vi "createQueryInputStr.vi"(8 "error in (no error)":errorcluster, 9 "CoolerQuery":T1=enum."ReadControlSensor", 11 "CoolerSerialCommand in":refnum<class "CoolerSerialCommand.lvclass">) -> (0 "error out":errorcluster, 2 "cmdDataStr":string, 3 "CoolerSerialCommand out":refnum<class "CoolerSerialCommand.lvclass">)   [LabVIEW 2016, in "CoolerSerialCommand.lvclass"]
uses:
  CoolerSerialCommand.lvclass
  typedefs/CoolerQuery.ctl
panel:
  out "length":i32
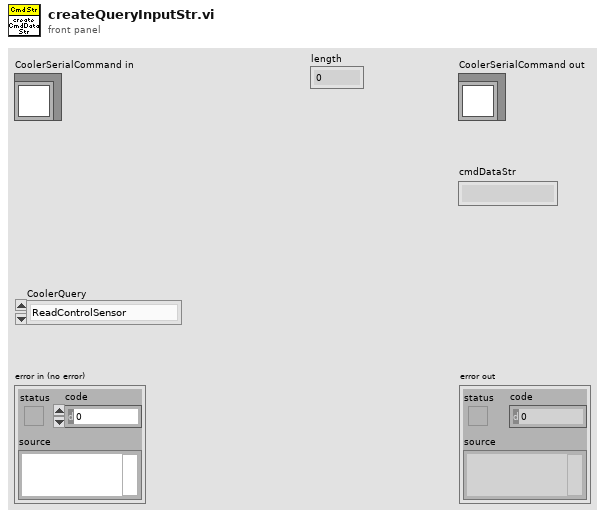
[diagram p1: front panel]
types:
  T1 = typedef "CoolerQuery.ctl" = enum16{"ReadSerialWatchdog", "ReadControlSensor", "ReadSetTemperature", "ReadSupplyTemperature", "ReadExternalRTD", "ReadExternalThermistor", "ReadReturnTemperature", "ReadAmbientTemperature", "ReadProcessFlow", "ReadTECBank1Current", "ReadTECBank2Current", "ReadTEDriveLevel", "ReadAlarmStateLevel1", "ReadAlarmStateLevel21", "ReadAlarmStateLevel22", "ReadWarningStateLevel1", "ReadHighSupplyTempWarning", "ReadLowSupplyTempWarning", "ReadHighAmbientTempWarning", "ReadLowAmbientTempWarning", "ReadLowProcessFlowWarning", "ReadHighSupplyTempAlarm", "ReadLowSupplyTempAlarm", "ReadHighAmbientTempAlarm", "ReadLowAmbientTempAlarm", "ReadLowProcessFlowAlarm", "ReadPWMandRelayStatus", "ReadPIDStatus", "ReadUnitUpTime", "ReadFan1Speed", "ReadFan2Speed", "ReadFan3Speed", "ReadFan4Speed"}
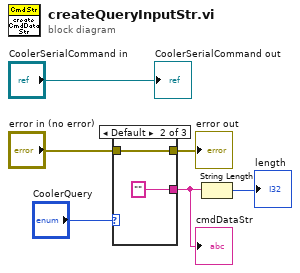
[diagram p0: block diagram]
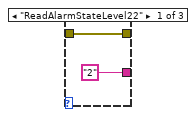
[diagram p2: hidden frame]
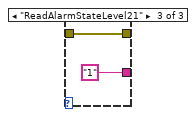
[diagram p3: hidden frame]
diagram:
  n1 = case shown="Default" "CoolerQuery" {
    tunnel: "error in (no error)" -> [w7 w10 w11]
    tunnel: ["2" "" "1"] -> w1
    tunnel: [w7 w10 w11] -> w2
    frame "ReadAlarmStateLevel22" {
    }
    frame Default {
    }
    frame "ReadAlarmStateLevel21" {
    }
  }
  "error out" <- w2
  "cmdDataStr" <- w1
  n2 = String Length(string=w1) -> (length=→"length":i32)
  "CoolerSerialCommand out" <- "CoolerSerialCommand in"
